vi "Update State Description (in Dictionary).vi"(8 "error in":errorcluster, 9 "description":string, 10 "state":string, 11 "routing channel in":T1 format="%.0x") -> (0 "error out":errorcluster, 3 "routing channel out":T1=18446744073709551615 format="%.0x")   [LabVIEW 2020, in "Routing and Faulting Scripting.lvlib"]
uses:
  Routing and Faulting Scripting.lvlib
  <vilib>/NI VeriStand/Custom Device API/Custom Device Item Ref.ctl
  NationalInstruments.VeriStand.SystemDefinitionAPI
  Constants/Scripting Constants.vi
  <vilib>/NI VeriStand/Custom Device API/Custom Device API.lvlib
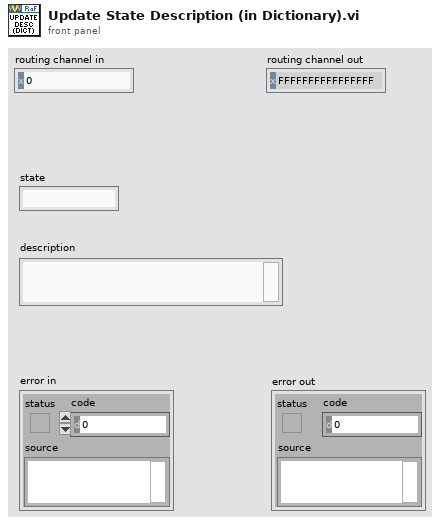
[diagram p1: front panel]
types:
  T1 = typedef "Custom Device API.lvlib/Custom Device Item Ref.ctl" = u64
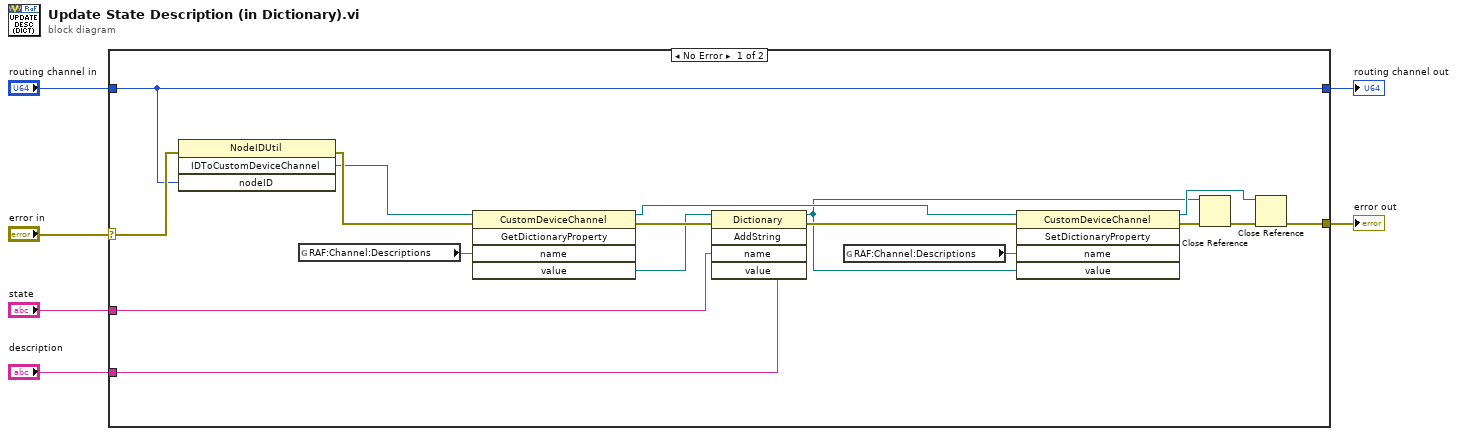
[diagram p0: block diagram]
diagram:
  n1 = case shown="No Error" "error in" {
    selector: "error in" -> [w23 w25]
    tunnel: [w7 w25] -> w5
    tunnel: "routing channel in" -> [w15 w24]
    tunnel: [w15 w24] -> w3
    tunnel: "state" -> [w14 _]
    tunnel: "description" -> [w13 _]
    frame No Error {
      n2 = invoke class="NodeIDUtil" method="IDToCustomDeviceChannel"(error in=w23, "nodeID"=w15) -> (error out=w19:errorcluster, "IDToCustomDeviceChannel"=w16:refnum<k24>)  [unwired: 2 in, 2 out]
      n3 = global read "Scripting Constants.vi" "RAF:Channel:Descriptions"() -> (w20:string)
      n4 = invoke class="CustomDeviceChannel" method="GetDictionaryProperty"(reference=w16, error in=w19, "name"=w20) -> (reference out=w12:refnum<k24>, error out=w18:errorcluster, "value"=w17:refnum<k24>)  [unwired: 2 in, 2 out]
      n5 = invoke class="Dictionary" method="AddString"(reference=w17, error in=w18, "name"=w14, "value"=w13) -> (reference out=w10:refnum<k24>, error out=w21:errorcluster)  [unwired: 1 in, 3 out]
      n6 = global read "Scripting Constants.vi" "RAF:Channel:Descriptions"() -> (w22:string)
      n7 = invoke class="CustomDeviceChannel" method="SetDictionaryProperty"(reference=w12, error in=w21, "name"=w22, "value"=w10) -> (reference out=w11:refnum<k24>, error out=w9:errorcluster)  [unwired: 1 in, 3 out]
      n8 = Close Reference(reference=w10, error in (no error)=w9) -> (error out=w8:errorcluster)
      n9 = Close Reference(reference=w11, error in (no error)=w8) -> (error out=w7:errorcluster)
    }
    frame Error {
    }
  }
  "routing channel out" <- w3
  "error out" <- w5
